vi "AuMT8852B Script Lock.vi"(5 "Lock state (Unlocked)":enum16{"Unlocked", "Locked"}(ring), 7 "Set/Get (Set)":enum16{"Set", "Get"}(ring), 8 "error in (no error)":errorcluster, 9 "Password (0)":i32, 10 "Script (3)":i32=3, 11 "VISA session":refnum<visa-resource-name>) -> (0 "error out":errorcluster, 2 "error code":i32, 3 "VISA session out":refnum<visa-resource-name>, 4 "Lock state out":enum16{"Unlocked", "Locked"}(ring))   [LabVIEW 2017]
doc: "Anritsu MT8852B Bluetooth Tester\n\nLocks or unlocks a script. A locked script cannot be modified.\n\nINPUTS\nSet/Get - whether the lock state is being changed or read.\nLock state - whether the script will be locked or unlocked.\nScript - which script is being locked or unlocked.\nPassword - required only when the lock state is being set.\n\nOUTPUTS\nLock state out - whether the script is currently locked or unlocked."
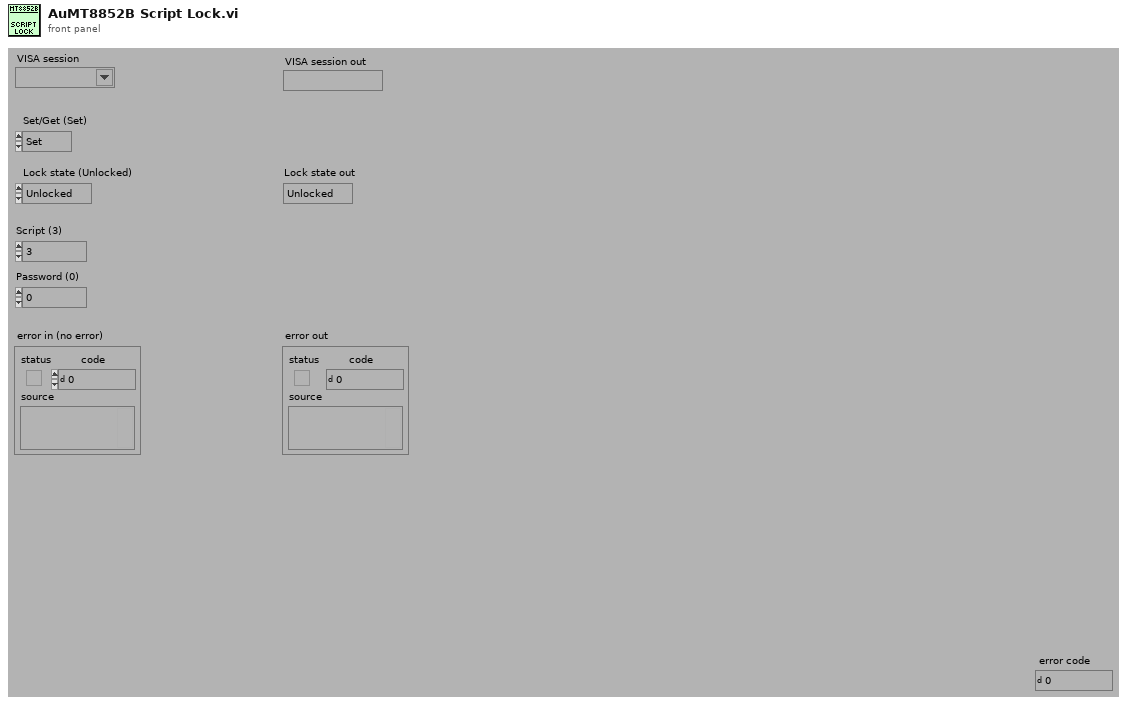
[diagram p1: front panel]
types:
  T1 = enum16{"Simulate", "Range check", "Cache", "Query instrument status"}
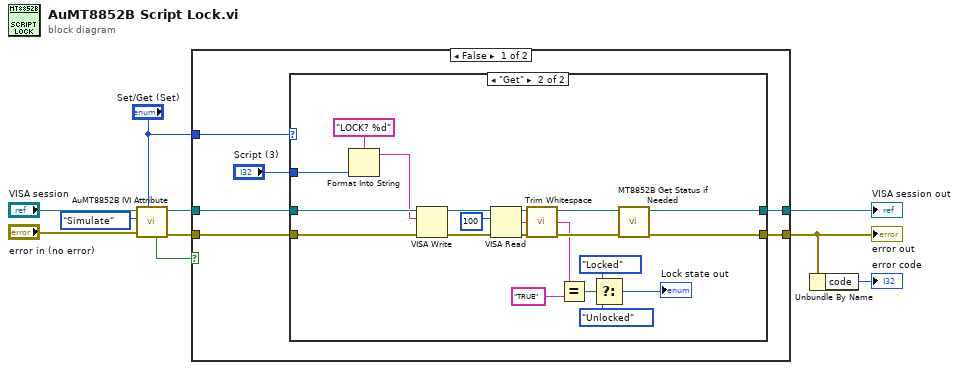
[diagram p0: block diagram]
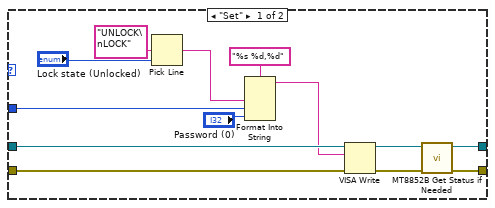
[diagram p2: hidden frame]
diagram:
  n1 = call <instrlib>:"AuMT8852B IVI Attribute.vi"("Set/Get (Set)"="Set/Get (Set)", "error in (no error)"="error in (no error)", "Flag (Simulate)"=T1."Simulate", "VISA session"="VISA session") -> ("error out"=w5:errorcluster, "VISA session out"=w7:refnum<visa-resource-name>, "Value out"=w4:bool)  [unwired: 5 in]
  n2 = case shown="False" w4 {
    tunnel: [w16 w50] -> w1
    tunnel: [w15 w49] -> w10
    tunnel: w7 -> [w14 w49]
    tunnel: w5 -> [w13 w50]
    tunnel: "Set/Get (Set)" -> [w12 _]
    frame False {
      n3 = case shown="\"Get\"" w12 {
        tunnel: [w29 w48] -> w16
        tunnel: [w28 w47] -> w15
        tunnel: w14 -> [w25 w46]
        tunnel: w13 -> [w24 w45]
        tunnel: "Script (3)" -> [w19 w42]
        frame "Set" {
          n4 = Pick Line(multi-line string="UNLOCK\nLOCK", line index="Lock state (Unlocked)") -> (output string=w20:string)  [unwired: 1 in]
          n5 = Format Into String(format string="%s %d,%d" ("Format String"), w20, w19, "Password (0)") -> (resulting string=w17:string)  [unwired: 2 in, 1 out]
          n6 = VISA Write(VISA resource name=w25, write buffer=w17, error in (no error)=w24) -> (VISA resource name out=w27:refnum<visa-resource-name>, error out=w26:errorcluster)  [unwired: 1 out]
          n7 = call <instrlib>:"MT8852B Get Status if Needed.vi"("error in (no error)"=w26, "VISA session"=w27) -> ("error out"=w29:errorcluster, "VISA session out"=w28:refnum<visa-resource-name>)  [unwired: 8 in]
        }
        frame "Get" {
          n8 = Format Into String(format string="LOCK? %d" ("Format String"), w42) -> (resulting string=w43:string)  [unwired: 2 in, 1 out]
          n9 = VISA Write(VISA resource name=w46, write buffer=w43, error in (no error)=w45) -> (VISA resource name out=w41:refnum<visa-resource-name>, error out=w40:errorcluster)  [unwired: 1 out]
          n10 = VISA Read(VISA resource name=w41, byte count=u32 100 ("byte count (0)"), error in (no error)=w40) -> (VISA resource name out=w39:refnum<visa-resource-name>, read buffer=w31:string, error out=w38:errorcluster)  [unwired: 1 out]
          n11 = call <vilib>:"Trim Whitespace.vi"("string"=w31) -> ("trimmed string"=w30:string)  [unwired: 1 in]
          n12 = Equal?(x=w30, y="TRUE") -> (x = y?=w36:bool)
          n13 = Select(t=enum16{"Unlocked", "Locked"}."Locked" ("Lock state (Unlocked)"), s=w36, f=enum16{"Unlocked", "Locked"}."Unlocked" ("Lock state (Unlocked)")) -> (s? t:f=→"Lock state out":enum16{"Unlocked", "Locked"})
          n14 = call <instrlib>:"MT8852B Get Status if Needed.vi"("error in (no error)"=w38, "VISA session"=w39) -> ("error out"=w48:errorcluster, "VISA session out"=w47:refnum<visa-resource-name>)  [unwired: 8 in]
        }
      }
    }
    frame True {
    }
  }
  "error out" <- w1
  "VISA session out" <- w10
  n15 = Unbundle By Name(w1) -> ("code"=→"error code":i32)
